vi "Kalman Filter.vi"(0 "Initial X Position Uncertainty (inch)":dbl format="%#_13g", 1 "Initial Y Position Uncertainty (inch)":dbl format="%#_13g", 2 "Initial Angle Uncertainty (degrees)":dbl format="%#_13g", 3 "Translate\nMotion?":bool=TRUE, 4 "Distance":dbl format="%#_13g", 5 "Wheel Angle":dbl format="%#_13g", 6 "Gyro Angle":dbl format="%#_13g", 7 "Magnetometer Angle":dbl format="%#_13g", 9 "Position Noise 1":dbl format="%#_13g", 10 "Magnetometer\nStd. Deviation":dbl=0.01 format="%#_13g", 13 "Position Noise 2":dbl format="%#_13g", 15 "Position Noise 3":dbl format="%#_13g", 16 "Gyro Angle\nStd. Deviation":dbl=0.01 format="%#_13g", 19 "Position Noise 4":dbl format="%#_13g") -> (20 "Robot Position Y":dbl, 23 "Robot Position X":dbl, 27 "Robot Heading Angle":dbl)   [LabVIEW 2014]
uses:
  <vilib>/Analysis/Matrix/Datatypes/RealMatrix.ctl
  <vilib>/Analysis/baseanly.llb/Real A x B.vi
  <vilib>/Analysis/7linalg.llb/Create Special Real Matrix.vi
  <vilib>/Analysis/Matrix/Numeric/Multiply/Multiply - RM,R.vi
  <vilib>/Analysis/Matrix/Numeric/Add/Add - RM,RM.vi
  <vilib>/Analysis/Matrix/Numeric/Add/Add (Elementwise) - RM,R.vi
  <vilib>/Analysis/Matrix/Numeric/Multiply/Multiply - RM,RM.vi
  <vilib>/Analysis/Matrix/Numeric/Subtract/Subtract - RM,RM.vi
  <vilib>/Analysis/Matrix/Numeric/Multiply/Multiply - R,RM.vi
  <vilib>/Analysis/NI_AALPro.lvlib
  <vilib>/Analysis/Matrix/NI_Matrix.lvlib
  <vilib>/Analysis/NI_AALBase.lvlib
panel:
  in  "stop":bool
  out "R":dbl
  out "K":T1
  in  "P- (k+1)":T1
  out "error 3":i32
  out "error 2":i32
  out "error":i32
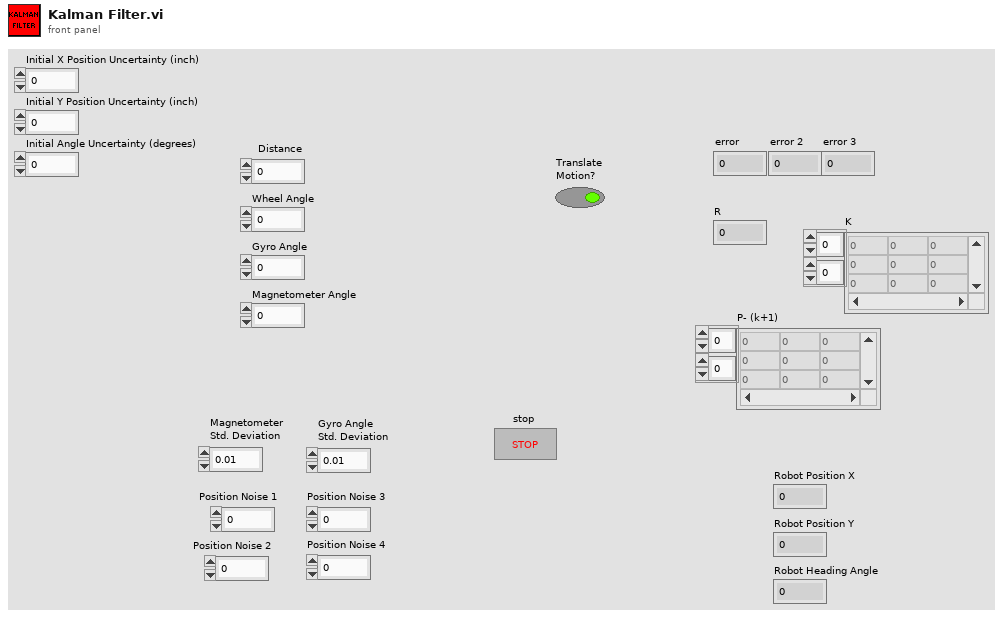
[diagram p1: front panel]
types:
  T1 = typedef "NI_Matrix.lvlib/RealMatrix.ctl" = dbl[][]
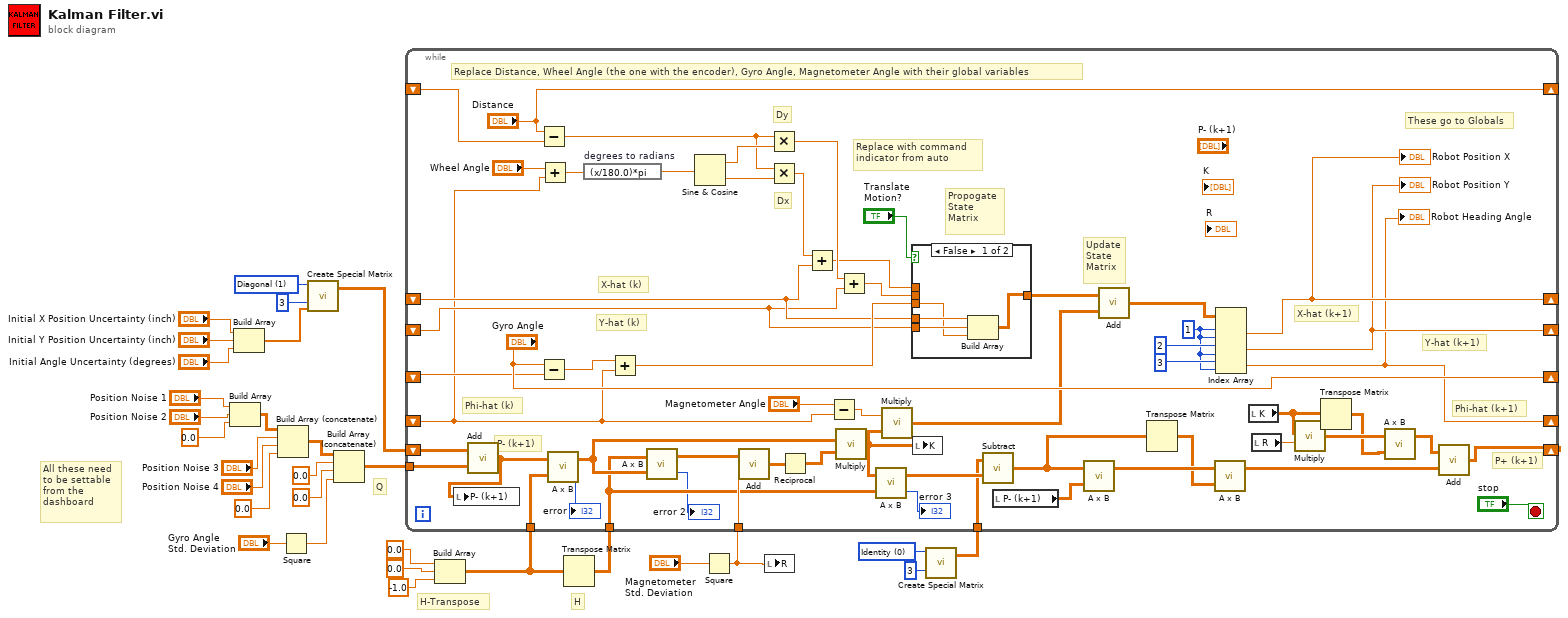
[diagram p0: block diagram]
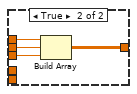
[diagram p2: hidden frame]
diagram:
  w7 = 1 items=["Identity", "Diagonal", "Toeplitz", "Vandermonde", "Companion", "Hankel", "Hadamard", "Wilkinson", "Hilbert", "Inverse Hilbert", "Rosser", "Pascal"] ("matrix type")
  w27 = 0 items=["Identity", "Diagonal", "Toeplitz", "Vandermonde", "Companion", "Hankel", "Hadamard", "Wilkinson", "Hilbert", "Inverse Hilbert", "Rosser", "Pascal"] ("matrix type")
  # "All these need \nto be settable\nfrom the\ndashboard"
  # "Q"
  # "H"
  # "H-Transpose"
  n1 = Build Array("Position Noise 1", "Position Noise 2", 0.0) -> (w21:T1)
  n2 = Build Array("Initial X Position Uncertainty (inch)", "Initial Y Position Uncertainty (inch)", "Initial Angle Uncertainty (degrees)") -> (w2:dbl[])
  n3 = Build Array (concatenate)(w21, "Position Noise 3", "Position Noise 4", 0.0) -> (w17:T1)
  n4 = Square(x="Gyro Angle\nStd. Deviation") -> (x^2=w14:dbl)
  n5 = call-poly <vilib>:"Create Special Matrix.vi"("matrix type"=w7, "matrix size"=3, "Input Vector1"=w2) -> ("Special Matrix"=w1:T1)  [unwired: 2 in, 1 out]
  n6 = Build Array (concatenate)(w17, 0.0, 0.0, w14) -> (w13:T1)
  n7 = Build Array(0.0, 0.0, -1.0) -> (w11:T1)
  n8 = Transpose Matrix(1:w11) -> (0:w12:T1)
  n9 = Square(x="Magnetometer\nStd. Deviation") -> (x^2=w8:dbl)
  n10 = local write "R"(w8) -> ()
  n11 = call-poly <vilib>:"Create Special Matrix.vi"("matrix type"=w27, "matrix size"=3) -> ("Special Matrix"=w9:T1)  [unwired: 3 in, 1 out]
  n12 = while {
    shift-right: ["Distance"] -> _
    shift-left: _ -> [w88]
    shift-right: ["Gyro Angle"] -> _
    shift-left: _ -> [w79]
    shift-right: [w31] -> _
    shift-left: _ -> [w63]
    shift-right: [w33] -> _
    shift-left: _ -> [w74]
    shift-right: [w32] -> _
    shift-left: _ -> [w73]
    shift-right: [w36] -> _
    shift-left: w1 -> [w35]
    tunnel: w13 -> [w70]
    tunnel: w12 -> [w55]
    tunnel: w11 -> [w69]
    tunnel: w8 -> [w67]
    tunnel: w9 -> [w50]
    stop <- "stop" stop-if-true
    w56 = 1 ("index (col)")
    # "These go to Globals"
    # "P+ (k+1)"
    # "Update\nState\nMatrix"
    # "P- (k+1)"
    # "Phi-hat (k)"
    # "Y-hat (k)"
    # "X-hat (k)"
    # "Replace with command\nindicator from auto"
    # "Propogate\nState\nMatrix"
    # "Y-hat (k+1)"
    # "X-hat (k+1)"
    # "Dx"
    # "Dy"
    # "Phi-hat (k+1)"
    # "Replace Distance, Wheel Angle (the one with the encoder), Gyro Angle, Magnetometer Angle with their global variables"
    n13 = call-poly <vilib>:"Add.vi"("Real Matrix B"=w70, "Real Matrix A"=w35) -> ("A + B"=w48:T1)
    n14 = local write "P- (k+1)"(w48) -> ()
    n15 = Subtract(x="Distance", y=w88) -> (x-y=w83:dbl)
    n16 = Subtract(x="Gyro Angle", y=w79) -> (x-y=w72:dbl)
    n17 = Add(x="Wheel Angle", y=w63) -> (x+y=w86:dbl)
    n18 = call-poly <vilib>:"A x B.vi"("B"=w69, "A"=w48) -> ("error"=→"error":i32, "A x B"=w66:T1)
    n19 = expression code="(x/180.0)*pi" "degrees to radians"(w86) -> (w85:dbl)
    n20 = Add(x=w72, y=w63) -> (x+y=w78:dbl)
    n21 = call-poly <vilib>:"A x B.vi"("B"=w66, "A"=w55) -> ("error"=→"error 2":i32, "A x B"=w68:T1)
    n22 = Sine & Cosine(0:w85) -> (1:w84:dbl, 2:w82:dbl)
    n23 = call-poly <vilib>:"Add.vi"("Real Scalar c"=w67, "Real Matrix A"=w68) -> ("A + c"=w49:T1)
    n24 = Multiply(x=w83, y=w84) -> (x*y=w80:dbl)
    n25 = Multiply(x=w83, y=w82) -> (x*y=w81:dbl)
    n26 = Reciprocal(x=w49) -> (1/x=w65:T1)
    n27 = Add(x=w81, y=w74) -> (x+y=w76:dbl)
    n28 = Subtract(x="Magnetometer Angle", y=w63) -> (x-y=w62:dbl)
    n29 = call-poly <vilib>:"Multiply.vi"("Real Matrix B"=w65, "Real Matrix A"=w66) -> ("A * B"=w43:T1)
    n30 = Add(x=w80, y=w73) -> (x+y=w77:dbl)
    n31 = call-poly <vilib>:"A x B.vi"("B"=w55, "A"=w43) -> ("error"=→"error 3":i32, "A x B"=w51:T1)
    n32 = call-poly <vilib>:"Multiply.vi"("Real Matrix A"=w43, "Real Scalar c"=w62) -> ("c * A"=w60:T1)
    n33 = case shown="False" "Translate\nMotion?" {
      tunnel: w78 -> [w91 w97]
      tunnel: w77 -> [_ w96]
      tunnel: w76 -> [_ w95]
      tunnel: w74 -> [w93 _]
      tunnel: w73 -> [w92 _]
      tunnel: [w90 w94] -> w61
      frame False {
        n34 = Build Array(w93, w92, w91) -> (w90:T1)
      }
      frame True {
        n35 = Build Array(w95, w96, w97) -> (w94:T1)
      }
    }
    n36 = local write "K"(w43) -> ()
    n37 = call-poly <vilib>:"Subtract.vi"("Real Matrix B"=w51, "Real Matrix A"=w50) -> ("A - B"=w46:T1)
    n38 = local read "P- (k+1)"() -> (w47:T1)
    n39 = call-poly <vilib>:"A x B.vi"("B"=w47, "A"=w46) -> ("A x B"=w45:T1)  [unwired: 1 out]
    n40 = call-poly <vilib>:"Add.vi"("Real Matrix B"=w60, "Real Matrix A"=w61) -> ("A + B"=w59:T1)
    n41 = Transpose Matrix(1:w46) -> (0:w44:T1)
    n42 = call-poly <vilib>:"A x B.vi"("B"=w44, "A"=w45) -> ("A x B"=w38:T1)  [unwired: 1 out]
    n43 = Index Array(array=w59, index (row) #1=w56, index (col) #1=w56, index (row) #2=2 ("index (row)"), index (col) #2=w56, index (row) #3=3 ("index (row)"), index (col) #3=w56) -> (element #1=w33:dbl, element #2=w32:dbl, element #3=w31:dbl)
    "Robot Position X" <- w33
    "Robot Position Y" <- w32
    "Robot Heading Angle" <- w31
    n44 = local read "K"() -> (w42:T1)
    n45 = local read "R"() -> (w41:dbl)
    n46 = call-poly <vilib>:"Multiply.vi"("Real Scalar c"=w41, "Real Matrix A"=w42) -> ("A * c"=w40:T1)
    n47 = Transpose Matrix(1:w42) -> (0:w39:T1)
    n48 = call-poly <vilib>:"A x B.vi"("B"=w39, "A"=w40) -> ("A x B"=w37:T1)  [unwired: 1 out]
    n49 = call-poly <vilib>:"Add.vi"("Real Matrix B"=w38, "Real Matrix A"=w37) -> ("A + B"=w36:T1)
  }
